vi "Analysis Workspace Execution Statistics.vi"(9 "Warmup Iterations":i32, 10 "Time Per Iteration 2":u32[](array[numeric]), 11 "Time Per Iteration":u32[](array[numeric])) -> (1 "Max Jitter":dbl, 2 "Mean Time":dbl, 3 "Execution Time":u32[][](array[numeric]), 4 "Max Jitter 2":dbl, 5 "Mean Time 2":dbl)   [LabVIEW 2023]
doc: "Calculate average execution time and maximum jitter for the VI running within the RT Analysis Workspace, and the VI running under normal execution."
uses:
  <vilib>/Analysis/NI_AALBase.lvlib
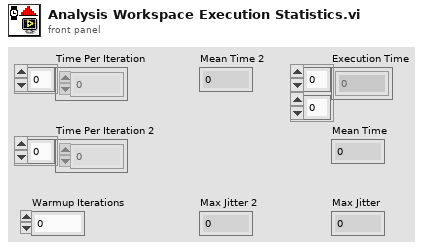
[diagram p1: front panel]
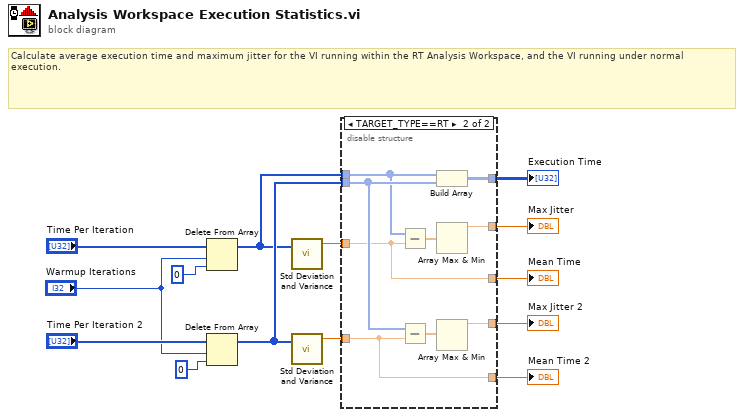
[diagram p0: block diagram]
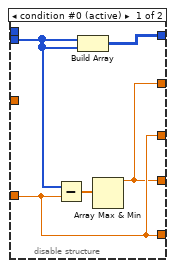
[diagram p2: hidden frame]
diagram:
  # "Calculate average execution time and maximum jitter for the VI running within the RT Analysis Workspace, and the VI running under normal execution."
  n1 = Delete From Array(array="Time Per Iteration", length="Warmup Iterations", index=0) -> (array with subset deleted=w3:u32[])  [unwired: 1 out]
  n2 = Delete From Array(array="Time Per Iteration 2", length="Warmup Iterations", index=0) -> (array with subset deleted=w4:u32[])  [unwired: 1 out]
  n3 = call <vilib>:"Std Deviation and Variance.vi"("X"=w3) -> ("mean"=w8:dbl)  [unwired: 1 in, 2 out]
  n4 = call <vilib>:"Std Deviation and Variance.vi"("X"=w4) -> ("mean"=w7:dbl)  [unwired: 1 in, 2 out]
  n5 = disable-structure shown="TARGET_TYPE==RT" {
    disable-tunnel: [w19 w28] -> w11
    disable-tunnel: [w15 w27] -> w10
    disable-tunnel: [w15 w26] -> w9
    disable-tunnel: w8 -> [_ w20]
    disable-tunnel: w7 -> [w16 w21]
    disable-tunnel: w4 -> [w17 w23]
    disable-tunnel: w3 -> [_ w22]
    disable-tunnel: [w16 w21] -> w2
    disable-tunnel: [w16 w20] -> w1
    frame condition #0 (active) {
      n6 = Subtract(x=w17, y=w16) -> (x-y=w18:dbl[])
      n7 = Build Array(w17, w17) -> (w19:u32[][])
      n8 = Array Max & Min(array=w18) -> (max value=w15:dbl)  [unwired: 3 out]
    }
    frame condition #1 {
      n9 = Subtract(x=w22, y=w20) -> (x-y=w25:dbl[])
      n10 = Subtract(x=w23, y=w21) -> (x-y=w24:dbl[])
      n11 = Build Array(w22, w23) -> (w28:u32[][])
      n12 = Array Max & Min(array=w25) -> (max value=w27:dbl)  [unwired: 3 out]
      n13 = Array Max & Min(array=w24) -> (max value=w26:dbl)  [unwired: 3 out]
    }
  }
  "Execution Time" <- w11
  "Mean Time" <- w1
  "Max Jitter" <- w10
  "Mean Time 2" <- w2
  "Max Jitter 2" <- w9
